vi "Deadzone.vi"(1 "Deadzone":dbl, 2 "Value":dbl) -> (0 "Numeric":dbl)   [LabVIEW 2016]
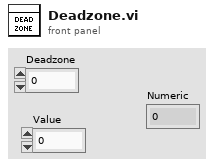
[diagram p1: front panel]
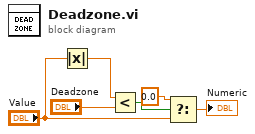
[diagram p0: block diagram]
diagram:
  n1 = Absolute Value(x="Value") -> (abs(x)=w4:dbl)
  n2 = Less?(x=w4, y="Deadzone") -> (x < y?=w5:bool)
  n3 = Select(t=0.0, s=w5, f="Value") -> (s? t:f=→"Numeric":dbl)
